vi "IntakeNetwork.vi"(8 "error in (no error)":errorcluster) -> (0 "error out":errorcluster)   [LabVIEW 2023]
doc: "Writes motor demand and sensor data to the Dashboard."
uses:
  IntakeGlobal.vi
  <vilib>/Rock Robotics/Network Tables/NT Write Boolean.vi
  <vilib>/Rock Robotics/Network Tables/NT Write Number.vi
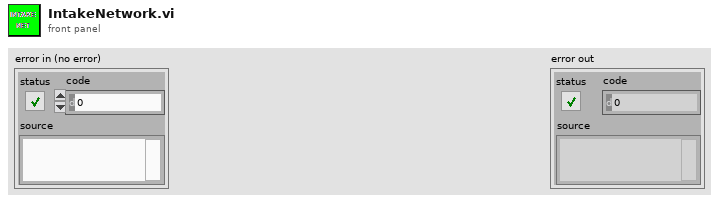
[diagram p1: front panel]
types:
  T1 = typedef "IntakeStates.ctl" = enum16{"Start", "WaitForCommand", "IntakeCoral", "IntakeAlgae", "WaitForCoral", "WaitForAlgae", "DepositCoral", "DepositAlgae", "DepositCoralTimer", "DepositAlgaeTimer"}
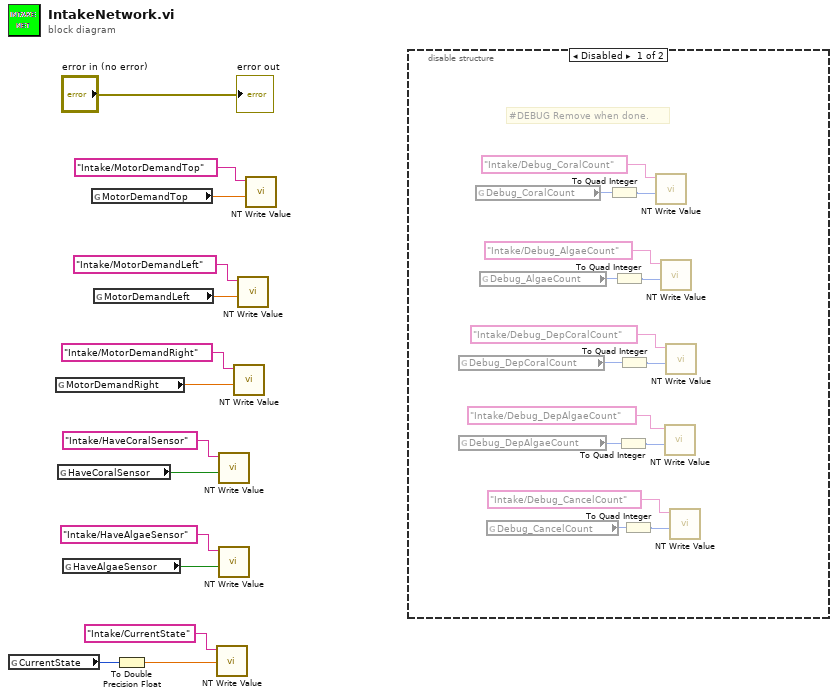
[diagram p0: block diagram]
diagram:
  n1 = global read "IntakeGlobal.vi" "CurrentState"() -> (w4:T1)
  n2 = global read "IntakeGlobal.vi" "MotorDemandRight"() -> (w7:dbl)
  n3 = global read "IntakeGlobal.vi" "HaveCoralSensor"() -> (w6:bool)
  n4 = global read "IntakeGlobal.vi" "HaveAlgaeSensor"() -> (w9:bool)
  n5 = global read "IntakeGlobal.vi" "MotorDemandTop"() -> (w1:dbl)
  n6 = global read "IntakeGlobal.vi" "MotorDemandLeft"() -> (w8:dbl)
  n7 = To Double Precision Float(number=w4) -> (double precision float=w3:dbl)
  n8 = call-poly <vilib>:"NT Write Value.vi"("value"=w3, "name"="Intake/CurrentState") -> ()  [unwired: 9 in, 1 out]
  n9 = call-poly <vilib>:"NT Write Value.vi"("value"=w6, "name"="Intake/HaveCoralSensor") -> ()  [unwired: 9 in, 1 out]
  n10 = call-poly <vilib>:"NT Write Value.vi"("value"=w9, "name"="Intake/HaveAlgaeSensor") -> ()  [unwired: 9 in, 1 out]
  n11 = call-poly <vilib>:"NT Write Value.vi"("value"=w7, "name"="Intake/MotorDemandRight") -> ()  [unwired: 9 in, 1 out]
  n12 = call-poly <vilib>:"NT Write Value.vi"("value"=w8, "name"="Intake/MotorDemandLeft") -> ()  [unwired: 9 in, 1 out]
  n13 = call-poly <vilib>:"NT Write Value.vi"("value"=w1, "name"="Intake/MotorDemandTop") -> ()  [unwired: 9 in, 1 out]
  n14 = disable-structure shown="Disabled" {
    frame Disabled {
      # "#DEBUG Remove when done."
      n15 = global read "IntakeGlobal.vi" "Debug_DepCoralCount"() -> (w21:i32)
      n16 = global read "IntakeGlobal.vi" "Debug_DepAlgaeCount"() -> (w19:i32)
      n17 = global read "IntakeGlobal.vi" "Debug_CoralCount"() -> (w27:i32)
      n18 = global read "IntakeGlobal.vi" "Debug_AlgaeCount"() -> (w24:i32)
      n19 = global read "IntakeGlobal.vi" "Debug_CancelCount"() -> (w16:i32)
      n20 = To Quad Integer(1:w27) -> (0:w28:i64)
      n21 = To Quad Integer(1:w24) -> (0:w25:i64)
      n22 = To Quad Integer(1:w19) -> (0:w20:i64)
      n23 = To Quad Integer(1:w21) -> (0:w22:i64)
      n24 = To Quad Integer(1:w16) -> (0:w17:i64)
      n25 = call-poly <vilib>:"NT Write Value.vi"("value"=w28, "name"="Intake/Debug_CoralCount") -> ()  [unwired: 9 in, 1 out]
      n26 = call-poly <vilib>:"NT Write Value.vi"("value"=w25, "name"="Intake/Debug_AlgaeCount") -> ()  [unwired: 9 in, 1 out]
      n27 = call-poly <vilib>:"NT Write Value.vi"("value"=w20, "name"="Intake/Debug_DepAlgaeCount") -> ()  [unwired: 9 in, 1 out]
      n28 = call-poly <vilib>:"NT Write Value.vi"("value"=w22, "name"="Intake/Debug_DepCoralCount") -> ()  [unwired: 9 in, 1 out]
      n29 = call-poly <vilib>:"NT Write Value.vi"("value"=w17, "name"="Intake/Debug_CancelCount") -> ()  [unwired: 9 in, 1 out]
    }
    frame Enabled {
    }
  }
  "error out" <- "error in (no error)"
